vi "表示法转换.vi"() -> ()   [LabVIEW 2023]
doc: "本VI是为《我和LabVIEW》一书编写的示例。\n关于本书的介绍请参考网页：\nhttp://ruanqizhen.spaces.live.com/blog/cns!5852D4F797C53FB6!4310.entry"
panel:
  in  "String":string
  out "U8 2":u8
  out "DBL result 2":dbl
  out "DBL result":dbl
  out "U8":u8
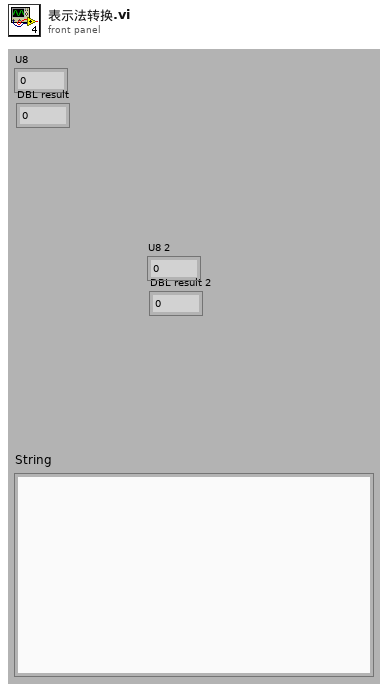
[diagram p1: front panel]
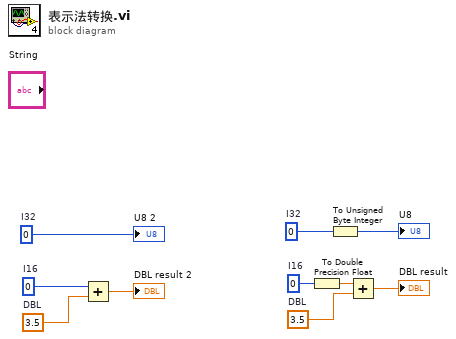
[diagram p0: block diagram]
diagram:
  w5 = 3.5  # DBL
  w4 = i16 0  # I16
  w3 = 0  # I32
  w8 = 3.5  # DBL
  w9 = i16 0  # I16
  w10 = 0  # I32
  n1 = Add(x=w4, y=w5) -> (x+y=→"DBL result 2":dbl)
  n2 = To Double Precision Float(number=w9) -> (double precision float=w1:dbl)
  n3 = To Unsigned Byte Integer(number=w10) -> (unsigned 8bit integer=→"U8":u8)
  n4 = Add(x=w1, y=w8) -> (x+y=→"DBL result":dbl)
  "U8 2" <- w3
